vi "SleepTime.vi"(2 "error in (no error)":errorcluster, 3 "Sleep":u32) -> (0 "error out":errorcluster)   [LabVIEW 2015]
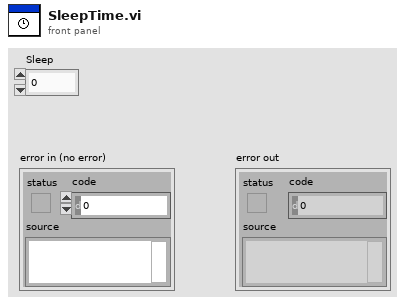
[diagram p1: front panel]
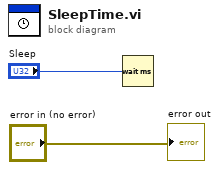
[diagram p0: block diagram]
diagram:
  n1 = Wait (ms)(milliseconds to wait="Sleep") -> ()  [unwired: 1 out]
  "error out" <- "error in (no error)"
